vi "Evaluate Partial Derivative.vi"(1 "Partial Index":i32, 2 "x=(x_1, ..., x_n)":dbl[](array[numeric]), 4 "Function Reference":refnum<vi>) -> (0 "df(x_1, ..., x_n)/dx_i":dbl)   [LabVIEW 2020, in "Automatic Differentiation.lvlib"]
doc: "Automatically evaluates the ith (where i is 0-indexed) partial derivative the given function at the value x = (x_1, ..., x_n). Only the function reference is required. The partial derivative is calculated automatically."
uses:
  Automatic Differentiation.lvlib
  classes/Dual/Dual.lvclass
  classes/Dual/Dual.lvclass/Dual.ctl
  49352e5e-86b6-4795-9dd0-b0f70ab2ee45.vi
  49352e5e-86b6-4795-9dd0-b0f70ab2ee45.vi/5957e011-cf56-4527-b6ed-13c3a4ca997b.vi
  classes/Dual/Write a.vi
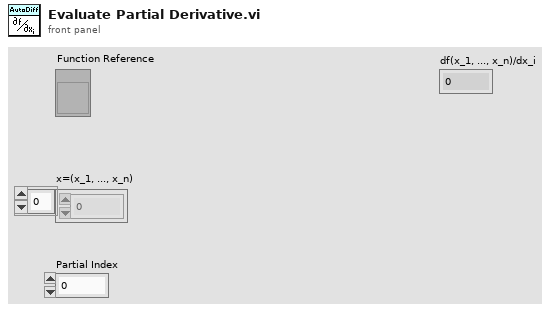
[diagram p1: front panel]
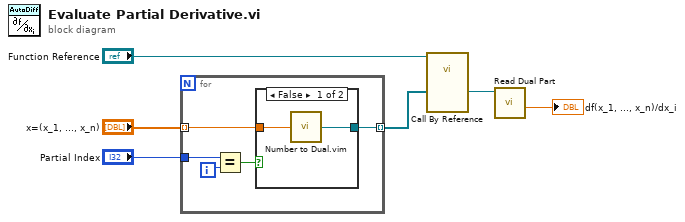
[diagram p0: block diagram]
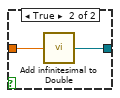
[diagram p2: hidden frame]
diagram:
  n1 = for {
    tunnel: "Partial Index" -> [w11]
    tunnel: "x=(x_1, ..., x_n)" -> [w9] mode=indexing
    tunnel: [w7] -> w3 mode=indexing
    i -> [w10]
    n2 = Equal?(x=w11, y=w10) -> (x = y?=w8:bool)
    n3 = case shown="False" w8 {
      tunnel: w9 -> [w13 w15]
      tunnel: [w12 w14] -> w7
      frame False {
        n4 = call "Number to Dual.vim"("Number"=w13) -> ("Dual"=w12:refnum<class "Dual.lvclass">)
      }
      frame True {
        n5 = call "Add infinitesimal to Double.vi"("DBL (x)"=w15) -> ("Dual (x+e)"=w14:refnum<class "Dual.lvclass">)
      }
    }
  }
  n6 = call-by-ref "?"(reference="Function Reference", "(x_1, ..., x_n)"=w3) -> ("f(x_1, ..., x_n)"=w2:refnum<class "Dual.lvclass">)  [unwired: 1 in, 2 out]
  n7 = call "Read Dual Part.vi"("Dual in"=w2) -> ("Dual Part"=→"df(x_1, ..., x_n)/dx_i":dbl)  [unwired: 9 in, 1 out]
